vi "HEWH Uniform Energy Factor Minimums.vi"(4 "Maufacturing Date":T7(ring), 7 "Water Heater Type":T6="Gas Storage (Non-Electric)", 8 "error in (no error)":errorcluster, 11 "UEF Calculated Values Input":T1 {"Data Indexes"."15 sec after Draw Index" format="%#.2f"; "Data Indexes"."15 sec after Draw Timestamp" format="%#.2f"; "Data Indexes"."Test Start Timestamp" format="%.2f"; "Data Indexes"."Test End Timestamp" format="%.2f"; "Data Indexes"."T0 Timestamp" format="%.2f"; "Data Indexes"."Tsf Timestamp" format="%.2f"; "Data Indexes"."Tsu0 Timestamp" format="%.2f"; "Data Indexes"."Tmax1 Timestamp" format="%.2f"; "Data Indexes"."Draw Index Timestamp" format="%#.2f"; "Data Indexes"."Non-Draw Timestamp" format="%#.2f"; "Data Indexes"."Heating Timestamp" format="%#.2f"; "Data Indexes"."Start Energy (BTU-Gas)" format="%.6f"; "Data Indexes"."Start Watt Hours" format="%.6f"; "Static Data"."V - Volume of Wh (True)" format="%.5f"; "Static Data"."T-Ambinet Nominal (°F)" format="%.5f"; "Static Data"."T-Inlet Setpoint (°F)" format="%.5f"; "Static Data"."T-Wh Setpoint (°F)" format="%.5f"; "Sampled Data"."Qe (Wh)" format="%.5f"; "Sampled Data"."Tau stby2 (hr)" format="%.5f"; "Sampled Data"."Tastby2 (°F)" format="%.5f"; "Sampled Data"."Qf (BTU)" format="%.5f"; "Sampled Data"."Qe (BTU)" format="%.5f"; "Sampled Data"."Tmax1 (°F)" format="%.5f"; "Sampled Data"."T0 (°F)" format="%.5f"; "Sampled Data"."Qr (BTU)" format="%.5f"; "Sampled Data"."T 24(°F)" format="%.5f"; "Sampled Data"."T astby(°F)" format="%.5f"; "Sampled Data"."T tstby(°F)" format="%.5f"; "Sampled Data"."T su0(°F)" format="%.5f"; "Sampled Data"."T suf(°F)" format="%.5f"; "Sampled Data"."Tau stby_1 (hr)" format="%.5f"; "Sampled Data"."Qsuf (BTU)" format="%.5f"; "Sampled Data"."Qsu0 (BTU)" format="%.5f"; "Calculated Values"."Draw Bonus Volume (gal)" format="%.6f"; "Calculated Values"."Adjustment Factor" format="%.6f"; "Calculated Values"."T*avg_del(n-1)" format="%.6f"; "Calculated Values"."T*min(n-1)" format="%.6f"; "Calculated Values"."T*avg_del(n)" format="%.6f"; "Calculated Values"."Vn" format="%.6f"; "Calculated Values"."Qdm (BTU)" format="%.6f"; "Calculated Values"."QHWD (BTU)" format="%.6f"; "Calculated Values"."QHW (BTU)" format="%.6f"; "Calculated Values"."UEF" format="%.6f"; "Calculated Values"."QHW67 (BTU)" format="%.6f"; "Calculated Values"."Qda (BTU)" format="%.6f"; "Calculated Values"."Qd (BTU)" format="%.6f"; "Calculated Values"."Q (BTU)" format="%.6f"; "Calculated Values"."UA (BTU/(hr*F))" format="%.6f"; "Calculated Values"."Qhr (BTU/hr)" format="%.6f"; "Calculated Values"."Qstby (BTU)" format="%.6f"; "Calculated Values"."nu_r" format="%.6f"; "Calculated Values"."CpUEF (BTU/(lb*F))" format="%.6f"; "Calculated Values"."rho_nu (lb/gal)" format="%.6f"; "Calculated Values"."V1- Vol (Gal)" format="%.6f"; "Calculated Values"."M cluster mass removed (lb)" format="%.6f"; "Calculated Values"."Cp theoretical (BTU/(lbm °F))" format="%.6f"; "Calculated Values"."Tin1 - Mean Inlet 1st Cluster (°F)" format="%.6f"; "Calculated Values"."Tdel1-Mean Outlet 1st Cluster(°F)" format="%.6f"; "Calculated Values"."Cp 24 (BTU/(lb*F))" format="%.6f"; "Calculated Values"."Cp standby (BTU/(lb*F))" format="%.6f"; "Calculated Values"."Cp2 (BTU/(lb*F))" format="%.6f"; "Calculated Values"."Cp1 (BTU/(lb*F))" format="%.6f"; "Calculated Values"."rho 24 (lb/gal)" format="%.6f"; "Calculated Values"."rho standby (lb/gal)" format="%.6f"; "Calculated Values"."rho 2 (lb/gal)" format="%.6f"; "Calculated Values"."Density of cold water All (lbm/gal)" format="%#.3g"; "Calculated Values"."CpHW (BTU/(lbm °F))" format="%#.3g"; "Calculated Values"."Density of hot water All (lbm/gal)" format="%#.3g"; "Calculated Values"."Mass of water All (lbm)" format="%#.3f"}) -> (0 "error out":errorcluster, 3 "UEF Calculated Values Output":T1 {"Data Indexes"."15 sec after Draw Index" format="%#.2f"; "Data Indexes"."15 sec after Draw Timestamp" format="%#.2f"; "Data Indexes"."Test Start Timestamp" format="%.2f"; "Data Indexes"."Test End Timestamp" format="%.2f"; "Data Indexes"."T0 Timestamp" format="%.2f"; "Data Indexes"."Tsf Timestamp" format="%.2f"; "Data Indexes"."Tsu0 Timestamp" format="%.2f"; "Data Indexes"."Tmax1 Timestamp" format="%.2f"; "Data Indexes"."Draw Index Timestamp" format="%#.2f"; "Data Indexes"."Non-Draw Timestamp" format="%#.2f"; "Data Indexes"."Heating Timestamp" format="%#.2f"; "Data Indexes"."Start Energy (BTU-Gas)" format="%.6f"; "Data Indexes"."Start Watt Hours" format="%.6f"; "Static Data"."V - Volume of Wh (True)" format="%.5f"; "Static Data"."T-Ambinet Nominal (°F)" format="%.5f"; "Static Data"."T-Inlet Setpoint (°F)" format="%.5f"; "Static Data"."T-Wh Setpoint (°F)" format="%.5f"; "Sampled Data"."Qe (Wh)" format="%.5f"; "Sampled Data"."Tau stby2 (hr)" format="%.5f"; "Sampled Data"."Tastby2 (°F)" format="%.5f"; "Sampled Data"."Qf (BTU)" format="%.5f"; "Sampled Data"."Qe (BTU)" format="%.5f"; "Sampled Data"."Tmax1 (°F)" format="%.5f"; "Sampled Data"."T0 (°F)" format="%.5f"; "Sampled Data"."Qr (BTU)" format="%.5f"; "Sampled Data"."T 24(°F)" format="%.5f"; "Sampled Data"."T astby(°F)" format="%.5f"; "Sampled Data"."T tstby(°F)" format="%.5f"; "Sampled Data"."T su0(°F)" format="%.5f"; "Sampled Data"."T suf(°F)" format="%.5f"; "Sampled Data"."Tau stby_1 (hr)" format="%.5f"; "Sampled Data"."Qsuf (BTU)" format="%.5f"; "Sampled Data"."Qsu0 (BTU)" format="%.5f"; "Calculated Values"."Draw Bonus Volume (gal)" format="%.6f"; "Calculated Values"."Adjustment Factor" format="%.6f"; "Calculated Values"."T*avg_del(n-1)" format="%.6f"; "Calculated Values"."T*min(n-1)" format="%.6f"; "Calculated Values"."T*avg_del(n)" format="%.6f"; "Calculated Values"."Vn" format="%.6f"; "Calculated Values"."Qdm (BTU)" format="%.6f"; "Calculated Values"."QHWD (BTU)" format="%.6f"; "Calculated Values"."QHW (BTU)" format="%.6f"; "Calculated Values"."UEF" format="%.6f"; "Calculated Values"."QHW67 (BTU)" format="%.6f"; "Calculated Values"."Qda (BTU)" format="%.6f"; "Calculated Values"."Qd (BTU)" format="%.6f"; "Calculated Values"."Q (BTU)" format="%.6f"; "Calculated Values"."UA (BTU/(hr*F))" format="%.6f"; "Calculated Values"."Qhr (BTU/hr)" format="%.6f"; "Calculated Values"."Qstby (BTU)" format="%.6f"; "Calculated Values"."nu_r" format="%.6f"; "Calculated Values"."CpUEF (BTU/(lb*F))" format="%.6f"; "Calculated Values"."rho_nu (lb/gal)" format="%.6f"; "Calculated Values"."V1- Vol (Gal)" format="%.6f"; "Calculated Values"."M cluster mass removed (lb)" format="%.6f"; "Calculated Values"."Cp theoretical (BTU/(lbm °F))" format="%.6f"; "Calculated Values"."Tin1 - Mean Inlet 1st Cluster (°F)" format="%.6f"; "Calculated Values"."Tdel1-Mean Outlet 1st Cluster(°F)" format="%.6f"; "Calculated Values"."Cp 24 (BTU/(lb*F))" format="%.6f"; "Calculated Values"."Cp standby (BTU/(lb*F))" format="%.6f"; "Calculated Values"."Cp2 (BTU/(lb*F))" format="%.6f"; "Calculated Values"."Cp1 (BTU/(lb*F))" format="%.6f"; "Calculated Values"."rho 24 (lb/gal)" format="%.6f"; "Calculated Values"."rho standby (lb/gal)" format="%.6f"; "Calculated Values"."rho 2 (lb/gal)" format="%.6f"; "Calculated Values"."Density of cold water All (lbm/gal)" format="%#.3g"; "Calculated Values"."CpHW (BTU/(lbm °F))" format="%#.3g"; "Calculated Values"."Density of hot water All (lbm/gal)" format="%#.3g"; "Calculated Values"."Mass of water All (lbm)" format="%#.3f"})   [LabVIEW 2023]
uses:
  Type Definitions/HEWH Water Heater Type.ctl
  Type Definitions/UEF Constants.ctl
  Type Definitions/HEWH Draw Stats.ctl
  Type Definitions/HEWH FHR Draw Type.ctl
  Type Definitions/FHR Bins.ctl
  Type Definitions/HEWH Meter Type.ctl
panel:
  # "FHR"
  # "FHR"
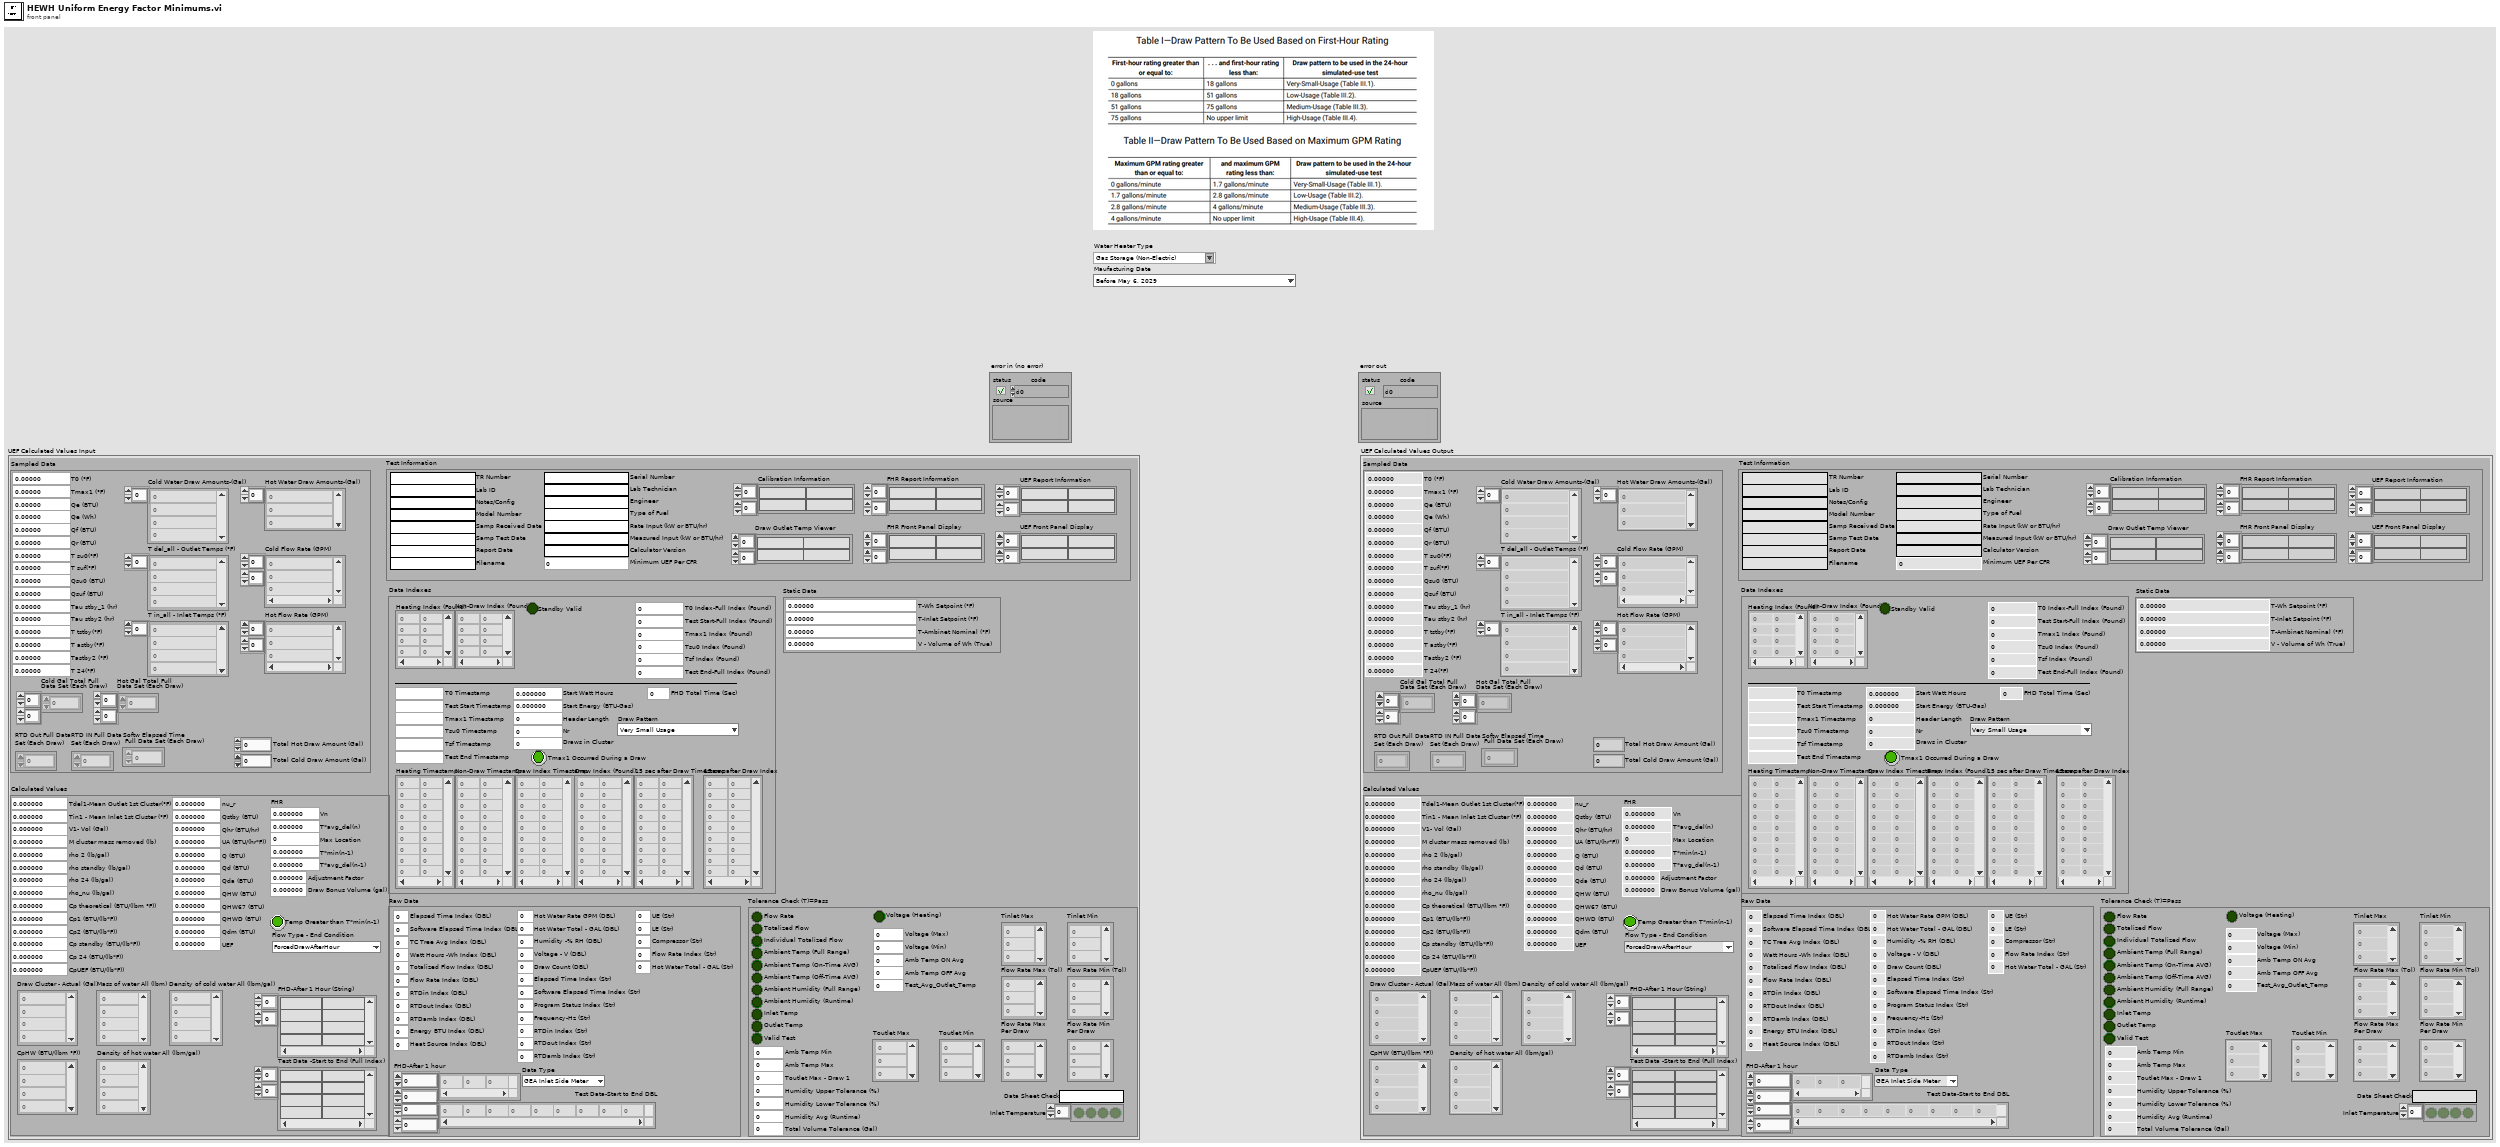
[diagram p1: front panel]
types:
  T1 = typedef "UEF Constants.ctl" = cluster{"Calculated Values":T2, "Sampled Data":cluster{"Cold Water Draw Amounts-(Gal)":dbl[], "T del_all - Outlet Temps (°F)":dbl[], "T in_all - Inlet Temps (°F)":dbl[], "Qsu0 (BTU)":dbl, "Qsuf (BTU)":dbl, "Tau stby_1 (hr)":dbl, "T suf(°F)":dbl, "T su0(°F)":dbl, "T tstby(°F)":dbl, "T astby(°F)":dbl, "T 24(°F)":dbl, "Qr (BTU)":dbl, "T0 (°F)":dbl, "Tmax1 (°F)":dbl, "Qe (BTU)":dbl, "Qf (BTU)":dbl, "Tastby2 (°F)":dbl, "RTD Out Full Data\nSet (Each Draw)":dbl[][], "RTD IN Full Data\nSet (Each Draw)":dbl[][], "Tau stby2 (hr)":dbl, "Hot Water Draw Amounts-(Gal)":dbl[], "Cold Flow Rate (GPM)":dbl[][], "Hot Flow Rate (GPM)":dbl[][], "Softw Elapsed Time\n Full Data Set (Each Draw)":dbl[][], "Cold Gal Total Full\nData Set (Each Draw)":dbl[][], "Total Hot Draw Amount (Gal) ":dbl, "Total Cold Draw Amount (Gal)":dbl, "Qe (Wh)":dbl, "Hot Gal Total Full\nData Set (Each Draw)":dbl[][]}, "Static Data":cluster{"T-Wh Setpoint (°F)":dbl, "T-Inlet Setpoint (°F)":dbl, "T-Ambinet Nominal (°F)":dbl, "V - Volume of Wh (True)":dbl}, "Data Indexes":cluster{"Test Start-Full Index (Found)":i32, "Header Length":i32, "Draw Index (Found)":i32[][], "Nr":i32, "Start Watt Hours":dbl, "Tsu0 Index (Found)":i32, "Tsf Index (Found)":i32, "Start Energy (BTU-Gas)":dbl, "Draws in Cluster":i32, "T0 Index-Full Index (Found)":i32, "Non-Draw Index (Found)":i32[][], "Tmax1 Index (Found)":i32, "Test End-Full Index (Found)":i32, "Heating Index (Found)":i32[][], "Heating Timestamp":dbl[][], "Non-Draw Timestamp":dbl[][], "Draw Index Timestamp":dbl[][], "Tmax1 Timestamp":dbl, "Tsu0 Timestamp":dbl, "Tsf Timestamp":dbl, "T0 Timestamp":dbl, "Test End Timestamp":dbl, "Test Start Timestamp":dbl, "15 sec after Draw Timestamp":dbl[][], "15 sec after Draw Index":dbl[][], "Tmax1 Occurred During a Draw":bool, "FHD Total Time (Sec)":dbl, "Draw Pattern":T4, "Standby Valid":bool}, "Raw Data":cluster{"Elapsed Time Index (DBL)":i32, "Software Elapsed Time Index (DBL)":i32, "TC Tree Avg Index (DBL)":i32, "Watt Hours -Wh Index (DBL)":i32, "Energy BTU Index (DBL)":i32, "Totalized Flow Index (DBL)":i32, "Flow Rate Index (DBL)":i32, "Program Status Index (Str)":i32, "RTDin Index (DBL)":i32, "RTDout Index (DBL)":i32, "RTDamb Index (DBL)":i32, "Test Data-Start to End DBL":dbl[][], "Data Type":T5, "Heat Source Index (DBL)":i32, "Hot Water Rate GPM (DBL)":i32, "Hot Water Total - GAL (DBL)":i32, "FHD-After 1 hour":dbl[][], "Humidity -% RH (DBL)":i32, "Voltage - V (DBL)":i32, "Draw Count (DBL)":i32, "Elapsed Time Index (Str)":i32, "Software Elapsed Time Index (Str)":i32, "Frequency-Hz (Str)":i32, "RTDin Index (Str)":i32, "RTDout Index (Str)":i32, "RTDamb Index (Str)":i32, "UE (Str)":i32, "LE (Str)":i32, "Compressor (Str)":i32, "Flow Rate Index (Str)":i32, "Hot Water Total - GAL (Str)":i32}, "Tolerance Check (T)=Pass":cluster{"Flow Rate":bool, "Totalized Flow":bool, "Ambient Temp (Full Range)":bool, "Ambient Humidity (Full Range)":bool, "Inlet Temp":bool, "Outlet Temp":bool, "Valid Test":bool, "Individual Totalized Flow":bool, "Data Sheet Check":string, "Inlet Temperature":bool[], "Tinlet Max":dbl[], "Tinlet Min":dbl[], "Flow Rate Max (Tol)":dbl[], "Flow Rate Min (Tol)":dbl[], "Amb Temp Max":dbl, "Amb Temp Min":dbl, "Toutlet Max - Draw 1":dbl, "Humidity Upper Tolerance (%)":dbl, "Total Volume Tolerance (Gal)":dbl, "Humidity Lower Tolerance (%)":dbl, "Flow Rate Max\nPer Draw":dbl[], "Flow Rate Min\nPer Draw":dbl[], "Ambient Humidity (Runtime)":bool, "Humidity Avg (Runtime)":dbl, "Ambient Temp (On-Time AVG)":bool, "Ambient Temp (Off-Time AVG)":bool, "Amb Temp OFF Avg":dbl, "Amb Temp ON Avg":dbl, "Voltage (Heating)":bool, "Voltage (Min)":dbl, "Voltage (Max)":dbl, "Toutlet Max":dbl[], "Toutlet Min":dbl[], "Test_Avg_Outlet_Temp":dbl}, "Test Information":cluster{"TR Number":string, "Lab ID":string, "Notes/Config":string, "Model Number":string, "Serial Number":string, "Lab Technician":string, "Engineer":string, "Type of Fuel":string, "Samp Received Date":string, "Samp Test Date":string, "Report Date":string, "Rate Input (kW or BTU/hr)":string, "Measured Input (kW or BTU/hr)":string, "Filename":string, "Calibration Information":string[][], "Calculator Version":string, "Minimum UEF Per CFR":dbl, "UEF Report Information":string[][], "FHR Report Information":string[][], "FHR Front Panel Display":string[][], "UEF Front Panel Display":string[][], "Draw Outlet Temp Viewer":string[][]}}
  T2 = typedef "HEWH Draw Stats.ctl" = cluster{"Draw Cluster - Actual (Gal)":dbl[], "Mass of water All (lbm)":dbl[], "Density of hot water All (lbm/gal)":dbl[], "CpHW (BTU/(lbm °F))":dbl[], "rho 2 (lb/gal)":dbl, "rho standby (lb/gal)":dbl, "rho 24 (lb/gal)":dbl, "Cp1 (BTU/(lb*F))":dbl, "Cp2 (BTU/(lb*F))":dbl, "Cp standby (BTU/(lb*F))":dbl, "Cp 24 (BTU/(lb*F))":dbl, "nu_r":dbl, "Qstby (BTU)":dbl, "Qhr (BTU/hr)":dbl, "UA (BTU/(hr*F))":dbl, "Q (BTU)":dbl, "Qd (BTU)":dbl, "Qda (BTU)":dbl, "QHW67 (BTU)":dbl, "UEF":dbl, "Tdel1-Mean Outlet 1st Cluster(°F)":dbl, "Tin1 - Mean Inlet 1st Cluster (°F)":dbl, "Cp theoretical (BTU/(lbm °F))":dbl, "M cluster mass removed (lb)":dbl, "V1- Vol (Gal)":dbl, "Test Data -Start to End (Full Index)":string[][], "rho_nu (lb/gal)":dbl, "Density of cold water All (lbm/gal)":dbl[], "CpUEF (BTU/(lb*F))":dbl, "QHW (BTU)":dbl, "QHWD (BTU)":dbl, "Qdm (BTU)":dbl, "FHD-After 1 Hour (String)":string[][], "Vn":dbl, "T*avg_del(n)":dbl, "Max Location":i32, "T*min(n-1)":dbl, "T*avg_del(n-1)":dbl, "Temp Greater than T*min(n-1)":bool, "Adjustment Factor":dbl, "Draw Bonus Volume (gal)":dbl, "Flow Type - End Condition":T3}
  T3 = typedef "HEWH FHR Draw Type.ctl" = enum16{"ForcedDrawAfterHour", "HeatingCutoffBeforeHour"}
  T4 = typedef "FHR Bins.ctl" = enum16{"Very Small Usage", "Low Usage", "Medium Usage", "High Usage", "Undefined"}
  T5 = typedef "HEWH Meter Type.ctl" = enum16{"GEA Inlet Side Meter", "GEA Outlet Side Meter", "CSA Inlet Side Meter"}
  T6 = typedef "HEWH Water Heater Type.ctl" = string
  T7 = enum16{"Before May 6, 2029", "On or After May 6, 2029"}
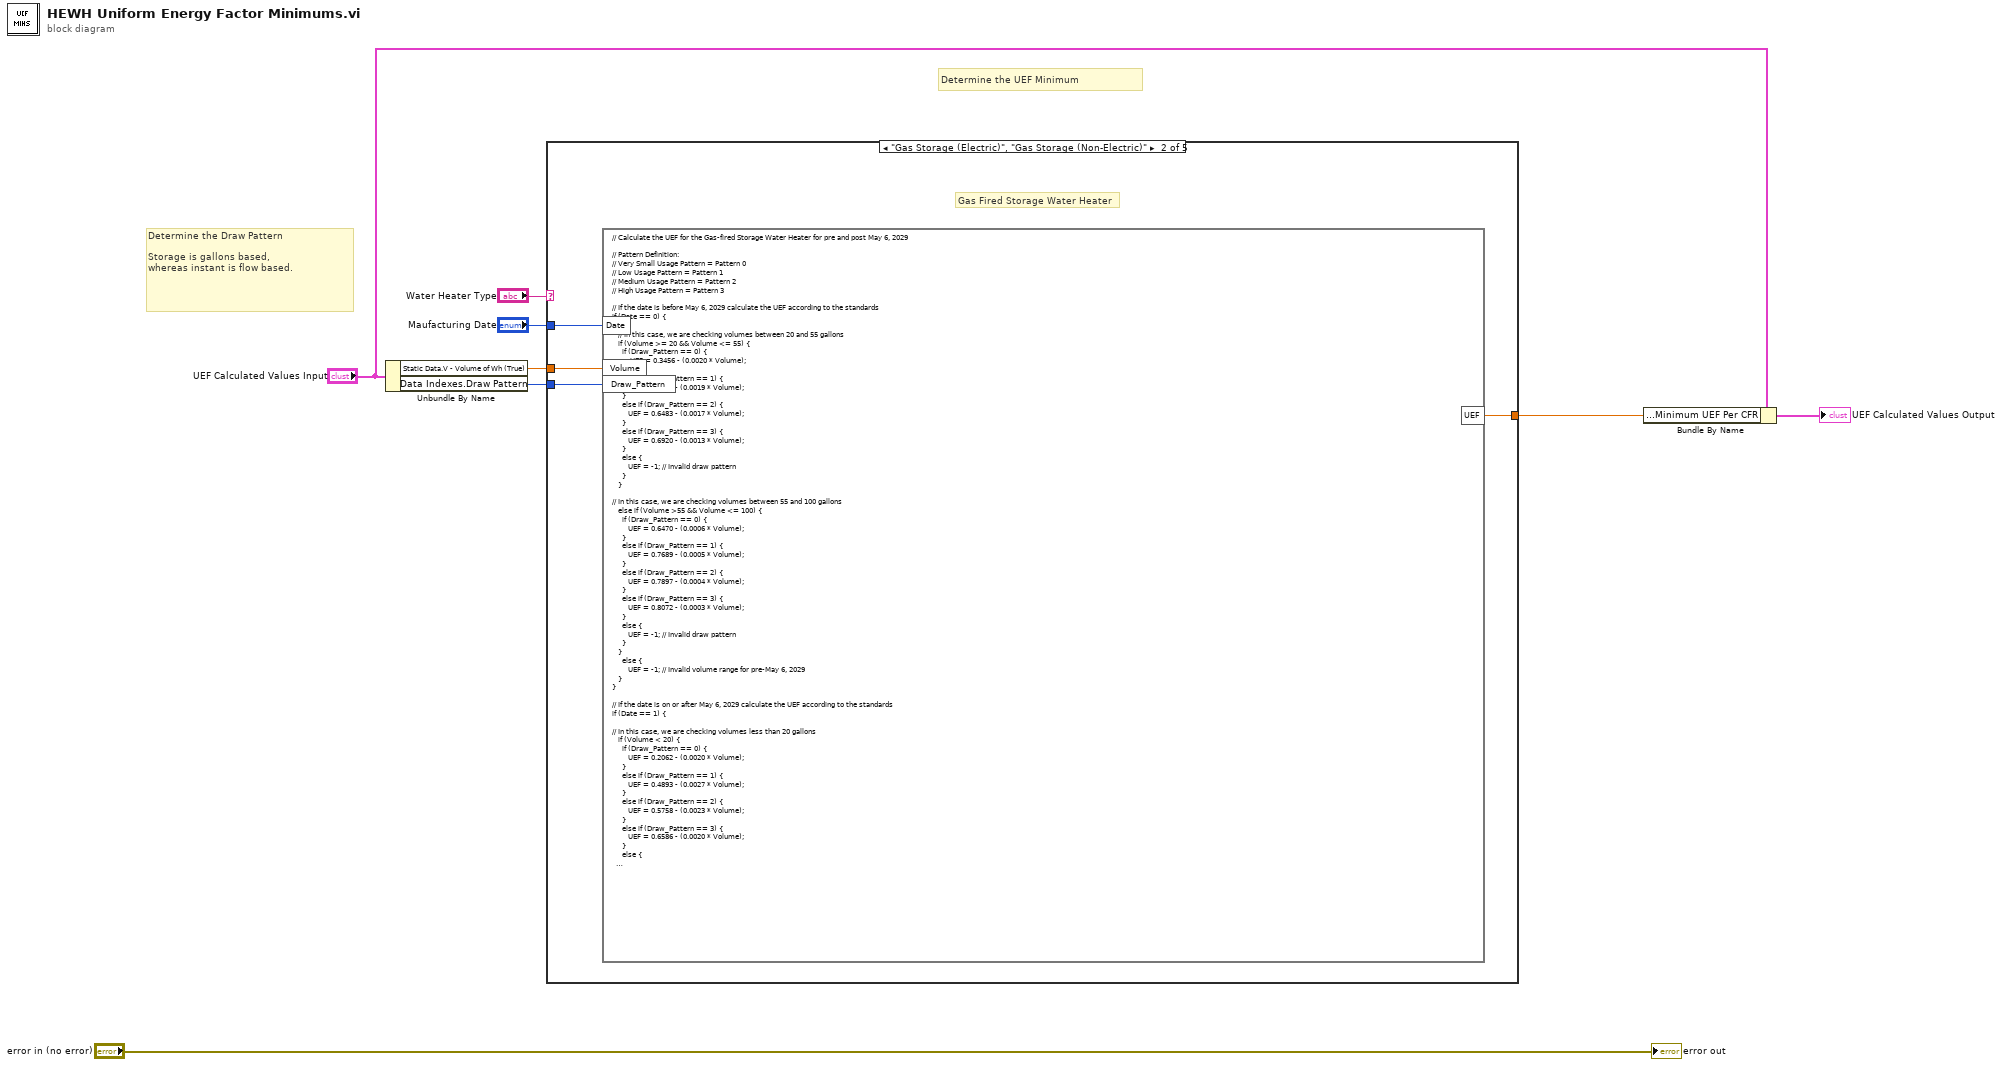
[diagram p0: block diagram]
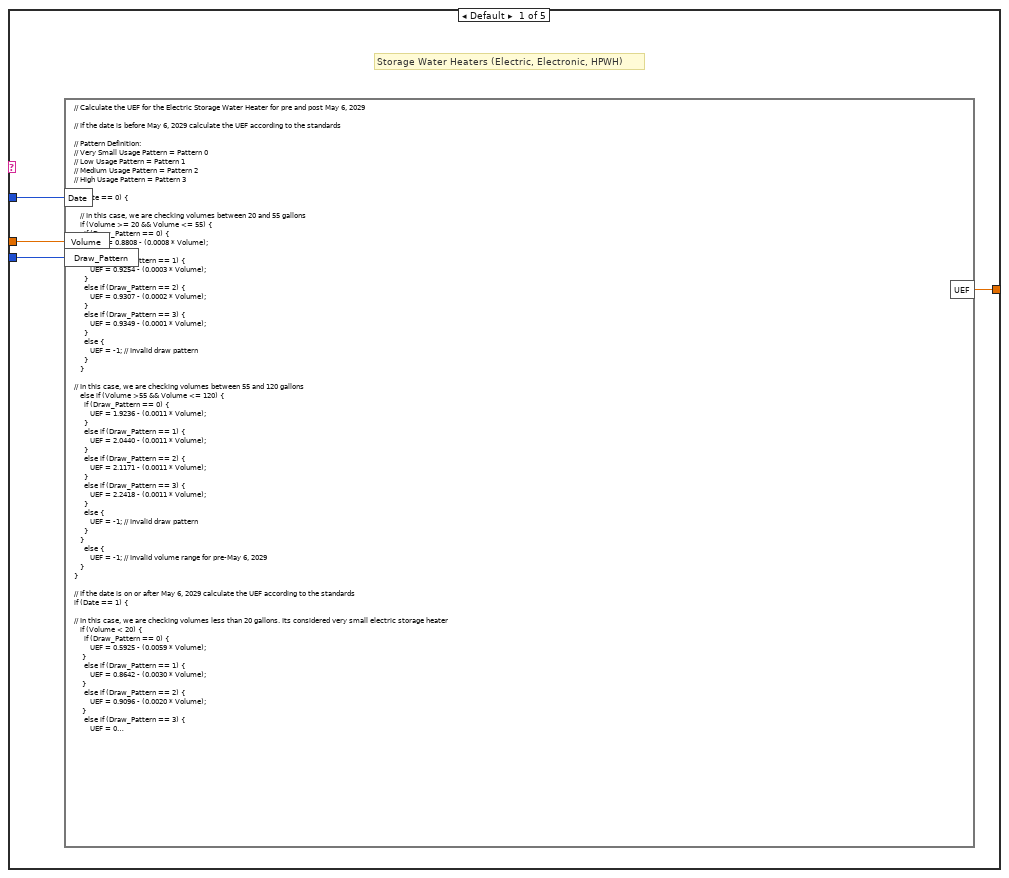
[diagram p2: hidden frame]
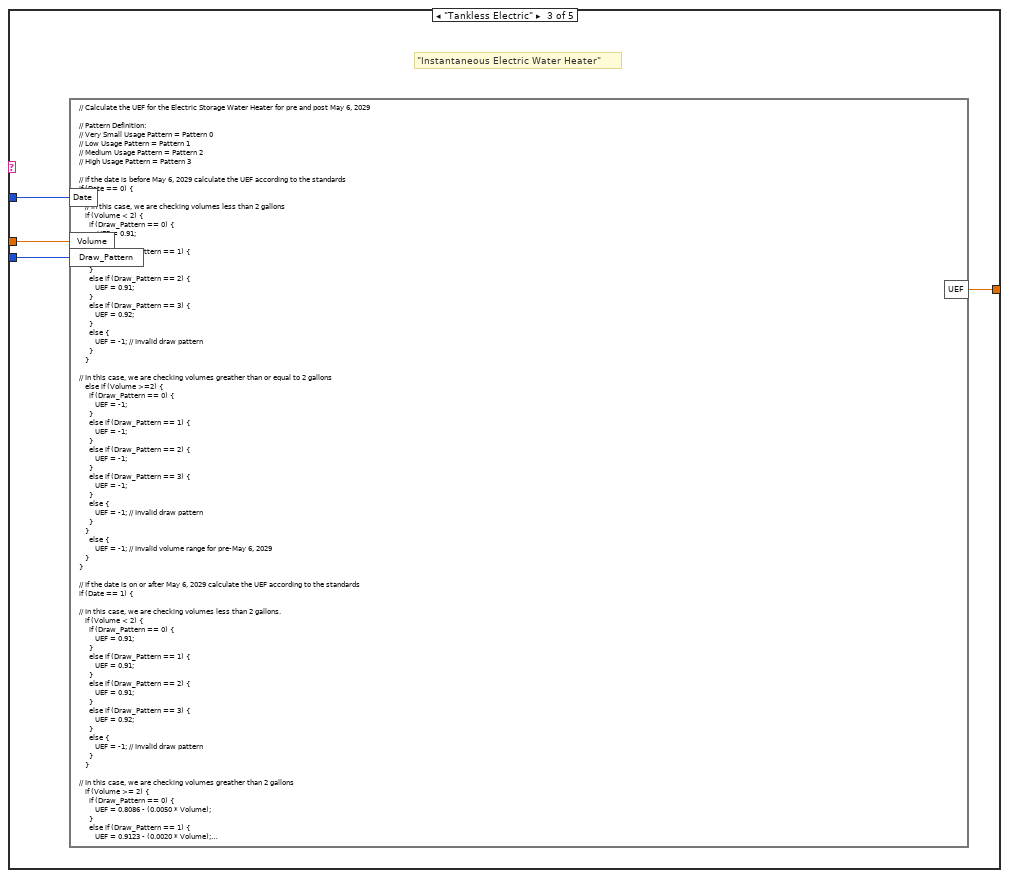
[diagram p3: hidden frame]
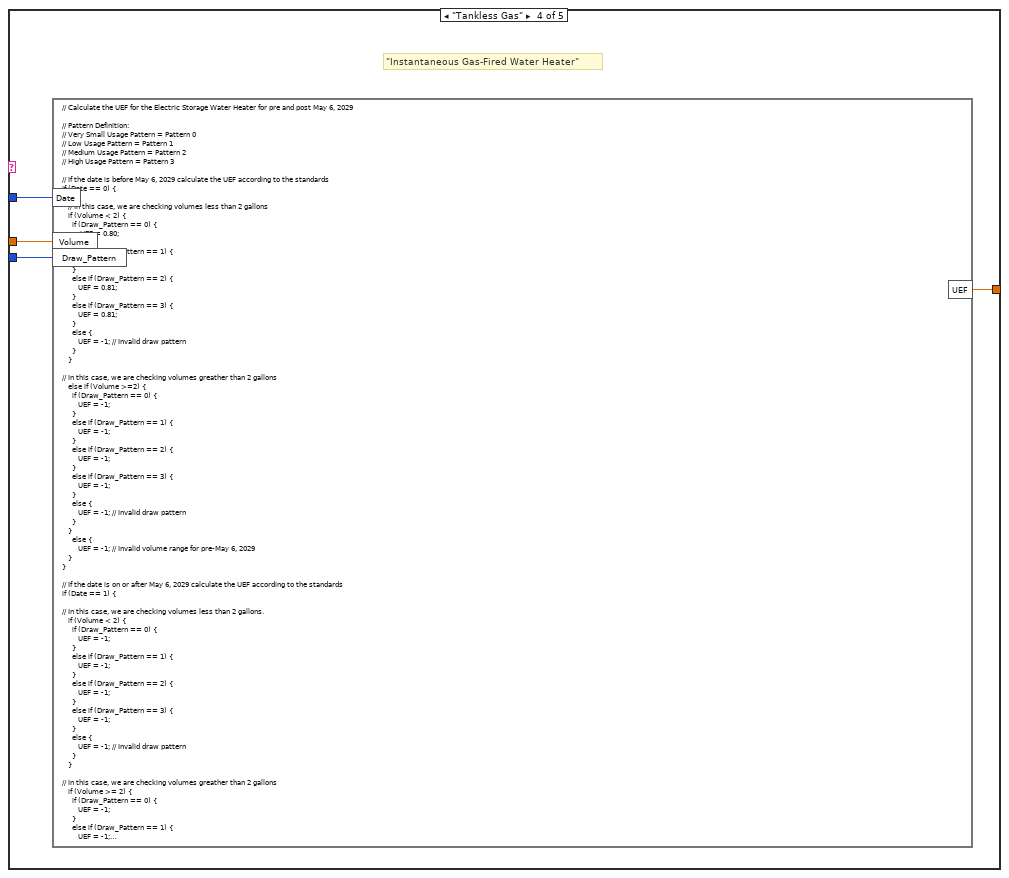
[diagram p4: hidden frame]
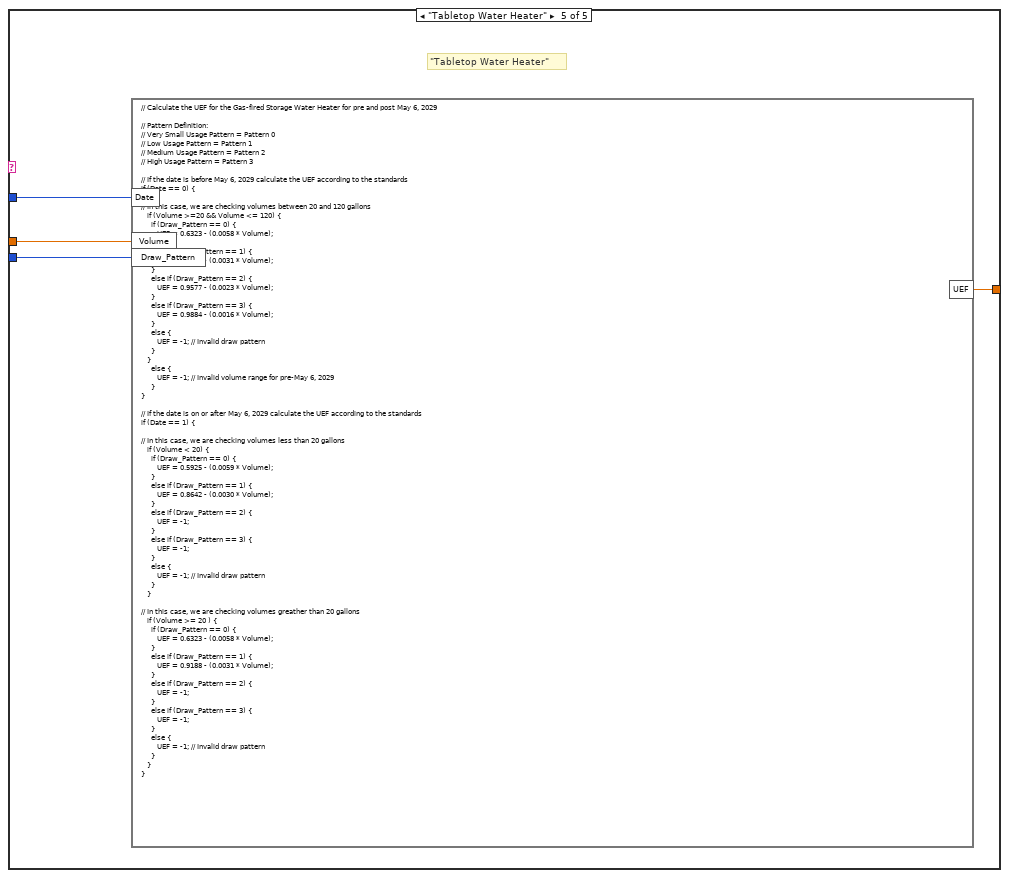
[diagram p5: hidden frame]
diagram:
  # "Determine the UEF Minimum"
  # "Determine the Draw Pattern\n\nStorage is gallons based,\nwhereas instant is flow based."
  n1 = Unbundle By Name("UEF Calculated Values Input") -> ("Static Data.V - Volume of Wh (True)"=w6:dbl, "Data Indexes.Draw Pattern"=w4:T4)
  n2 = case shown="\"Gas Storage (Electric)\", \"Gas Storage (Non-Electric)\"" "Water Heater Type" {
    tunnel: w6 -> [w9 w16 w19 w23 w27]
    tunnel: w4 -> [w10 w15 w18 w22 w26]
    tunnel: [w12 w14 w20 w24 w28] -> w1
    tunnel: "Maufacturing Date" -> [w11 w13 w17 w21 w25]
    frame Default {
      # "Storage Water Heaters (Electric, Electronic, HPWH)"
      n3 = formula code="// Calculate the UEF for the Electric Storage Water Heater for pre and post May 6, 2029\n\n// If the date is before May 6, 2029 calculate the UEF according to the standards\n\n// Pattern Definition:\n// Very Small Usage Pattern = Pattern 0\n// Low Usage Pattern = Pattern 1\n// Medium Usage Pattern = Pattern 2\n// High Usage Pattern = Pattern 3\n\nif (Date == 0) {\n\n   // In this case, we are checking volumes between 20 and 55 gallons\n   if (Volume >= 20 && Volume <= 55) {\n     if (Draw_Pattern == 0) {\n         UEF = 0.8808 - (0.0008 * Volume);\n     } \n     else if (Draw_Pattern == 1) {\n        UEF = 0.9254 - (0.0003 * Volume);\n     } \n     else if (Draw_Pattern == 2) {\n        UEF = 0.9307 - (0.0002 * Volume);\n     } \n     else if (Draw_Pattern == 3) {\n        UEF = 0.9349 - (0.0001 * Volume);\n     }\n     else {\n        UEF = -1; // Invalid draw pattern\n     }\n   } \n\n// In this case, we are checking volumes between 55 and 120 gallons\n   else if (Volume >55 && Volume <= 120) {\n     if (Draw_Pattern == 0) {\n        UEF = 1.9236 - (0.0011 * Volume);\n     } \n     else if (Draw_Pattern == 1) {\n        UEF = 2.0440 - (0.0011 * Volume);\n     } \n     else if (Draw_Pattern == 2) {\n        UEF = 2.1171 - (0.0011 * Volume);\n     } \n     else if (Draw_Pattern == 3) {\n        UEF = 2.2418 - (0.0011 * Volume);\n     }\n     else {\n        UEF = -1; // Invalid draw pattern\n     }\n   }\n     else {\n        UEF = -1; // Invalid volume range for pre-May 6, 2029\n   } \n}\n\n// If the date is on or after May 6, 2029 calculate the UEF according to the standards\nif (Date == 1) {\n\n// In this case, we are checking volumes less than 20 gallons. Its considered very small electric storage heater\n   if (Volume < 20) {\n     if (Draw_Pattern == 0) {\n        UEF = 0.5925 - (0.0059 * Volume);\n    } \n     else if (Draw_Pattern == 1) {\n        UEF = 0.8642 - (0.0030 * Volume);\n    } \n     else if (Draw_Pattern == 2) {\n        UEF = 0.9096 - (0.0020 * Volume);\n    } \n     else if (Draw_Pattern == 3) {\n        UEF = 0.9430 - (0.0012 * Volume);\n    }\n     else {\n        UEF = -1; // Invalid draw pattern\n    }\n}\n\n// In this case, we are checking volumes between 20 and 55 gallons, not considered small electric water heater)\n   if (Volume >= 20 && Volume <= 55) {\n     if (Draw_Pattern == 0) {\n        UEF = 2.30;\n    } \n     else if (Draw_Pattern == 1) {\n        UEF = 2.30;\n    } \n     else if (Draw_Pattern == 2) {\n        UEF = 2.30;\n    } \n     else if (Draw_Pattern == 3) {\n        UEF = 2.30;\n    }\n     else {\n        UEF = -1; // Invalid draw pattern\n    }\n} \n\n// In this case, we are checking volumes between 55 and 120 gallons\n   if (Volume >55 && Volume <= 120) {\n     if (Draw_Pattern == 0) {\n        UEF = 2.50;\n    } \n     else if (Draw_Pattern == 1) {\n        UEF = 2.50;\n    } \n     else if (Draw_Pattern == 2) {\n        UEF = 2.50;\n    } \n     else if (Draw_Pattern == 3) {\n        UEF = 2.50;\n    }\n     else {\n        UEF = -1; // Invalid draw pattern\n    }\n} \n\n// In this case, we are checking volumes greater than 120 gallons\n   if (Volume > 120) {\n     if (Draw_Pattern == 0) {\n        UEF = 0.3574 - (0.0012 * Volume);\n    } \n     else if (Draw_Pattern == 1) {\n        UEF = 0.7897 - (0.0019 * Volume);\n    } \n     else if (Draw_Pattern == 2) {\n        UEF = 0.8884 - (0.0017 * Volume);\n    } \n     else if (Draw_Pattern == 3) {\n        UEF = 0.9575 - (0.0013 * Volume);\n    }\n     else {\n        UEF = -1; // Invalid draw pattern\n    }\n}\n}"("Volume"=w9, "Draw_Pattern"=w10, "Date"=w11) -> ("UEF"=w12:dbl)
    }
    frame "Gas Storage (Electric)", "Gas Storage (Non-Electric)" {
      # "Gas Fired Storage Water Heater"
      n4 = formula code="// Calculate the UEF for the Gas-fired Storage Water Heater for pre and post May 6, 2029\n\n// Pattern Definition:\n// Very Small Usage Pattern = Pattern 0\n// Low Usage Pattern = Pattern 1\n// Medium Usage Pattern = Pattern 2\n// High Usage Pattern = Pattern 3\n\n// If the date is before May 6, 2029 calculate the UEF according to the standards\nif (Date == 0) {\n\n   // In this case, we are checking volumes between 20 and 55 gallons\n   if (Volume >= 20 && Volume <= 55) {\n     if (Draw_Pattern == 0) {\n         UEF = 0.3456 - (0.0020 * Volume);\n     } \n     else if (Draw_Pattern == 1) {\n        UEF = 0.5982 - (0.0019 * Volume);\n     } \n     else if (Draw_Pattern == 2) {\n        UEF = 0.6483 - (0.0017 * Volume);\n     } \n     else if (Draw_Pattern == 3) {\n        UEF = 0.6920 - (0.0013 * Volume);\n     }\n     else {\n        UEF = -1; // Invalid draw pattern\n     }\n   } \n\n// In this case, we are checking volumes between 55 and 100 gallons\n   else if (Volume >55 && Volume <= 100) {\n     if (Draw_Pattern == 0) {\n        UEF = 0.6470 - (0.0006 * Volume);\n     } \n     else if (Draw_Pattern == 1) {\n        UEF = 0.7689 - (0.0005 * Volume);\n     } \n     else if (Draw_Pattern == 2) {\n        UEF = 0.7897 - (0.0004 * Volume);\n     } \n     else if (Draw_Pattern == 3) {\n        UEF = 0.8072 - (0.0003 * Volume);\n     }\n     else {\n        UEF = -1; // Invalid draw pattern\n     }\n   }\n     else {\n        UEF = -1; // Invalid volume range for pre-May 6, 2029\n   } \n}\n\n// If the date is on or after May 6, 2029 calculate the UEF according to the standards\nif (Date == 1) {\n\n// In this case, we are checking volumes less than 20 gallons\n   if (Volume < 20) {\n     if (Draw_Pattern == 0) {\n        UEF = 0.2062 - (0.0020 * Volume);\n     } \n     else if (Draw_Pattern == 1) {\n        UEF = 0.4893 - (0.0027 * Volume);\n     } \n     else if (Draw_Pattern == 2) {\n        UEF = 0.5758 - (0.0023 * Volume);\n     } \n     else if (Draw_Pattern == 3) {\n        UEF = 0.6586 - (0.0020 * Volume);\n     }\n     else {\n        UEF = -1; // Invalid draw pattern\n     }\n   }\n\n// In this case, we are checking volumes between 20 and 55 gallons\n   if (Volume >= 20 && Volume <= 55) {\n     if (Draw_Pattern == 0) {\n        UEF = 0.3925 - (0.0020 * Volume);\n     } \n     else if (Draw_Pattern == 1) {\n        UEF = 0.6451 - (0.0019 * Volume);\n     } \n     else if (Draw_Pattern == 2) {\n        UEF = 0.7046 - (0.0017 * Volume);\n     } \n     else if (Draw_Pattern == 3) {\n        UEF = 0.7424 - (0.0013 * Volume);\n     }\n     else {\n        UEF = -1; // Invalid draw pattern\n     }\n   } \n\n// In this case, we are checking volumes between 55 and 100 gallons\n   if (Volume >55 && Volume <= 100) {\n     if (Draw_Pattern == 0) {\n        UEF = 0.6470 - (0.0006 * Volume);\n     } \n     else if (Draw_Pattern == 1) {\n        UEF = 0.7689 - (0.0005 * Volume);\n     } \n     else if (Draw_Pattern == 2) {\n        UEF = 0.7897 - (0.0004 * Volume);\n     } \n     else if (Draw_Pattern == 3) {\n        UEF = 0.8072 - (0.0003 * Volume);\n     }\n     else {\n        UEF = -1; // Invalid draw pattern\n     }\n   } \n\n// In this case, we are checking volumes greater than 100 gallons\n   if (Volume > 100) {\n     if (Draw_Pattern == 0) {\n        UEF = 0.1482 - (0.0007 * Volume);\n     } \n     else if (Draw_Pattern == 1) {\n        UEF = 0.4342 - (0.0017 * Volume);\n     } \n     else if (Draw_Pattern == 2) {\n        UEF = 0.5596 - (0.0020 * Volume);\n     } \n     else if (Draw_Pattern == 3) {\n        UEF = 0.6658 - (0.0019 * Volume);\n     }\n     else {\n        UEF = -1; // Invalid draw pattern\n     }\n   }\n}"("Volume"=w16, "Draw_Pattern"=w15, "Date"=w13) -> ("UEF"=w14:dbl)
    }
    frame "Tankless Electric" {
      # "\"Instantaneous Electric Water Heater\""
      n5 = formula code="// Calculate the UEF for the Electric Storage Water Heater for pre and post May 6, 2029\n\n// Pattern Definition:\n// Very Small Usage Pattern = Pattern 0\n// Low Usage Pattern = Pattern 1\n// Medium Usage Pattern = Pattern 2\n// High Usage Pattern = Pattern 3\n\n// If the date is before May 6, 2029 calculate the UEF according to the standards\nif (Date == 0) {\n\n   // In this case, we are checking volumes less than 2 gallons\n   if (Volume < 2) {\n     if (Draw_Pattern == 0) {\n         UEF = 0.91;\n     } \n     else if (Draw_Pattern == 1) {\n        UEF = 0.91;\n     } \n     else if (Draw_Pattern == 2) {\n        UEF = 0.91;\n     } \n     else if (Draw_Pattern == 3) {\n        UEF = 0.92;\n     }\n     else {\n        UEF = -1; // Invalid draw pattern\n     }   \n   } \n\n// In this case, we are checking volumes greather than or equal to 2 gallons\n   else if (Volume >=2) {\n     if (Draw_Pattern == 0) {\n        UEF = -1;\n     } \n     else if (Draw_Pattern == 1) {\n        UEF = -1;\n     } \n     else if (Draw_Pattern == 2) {\n        UEF = -1;\n     } \n     else if (Draw_Pattern == 3) {\n        UEF = -1;\n     }\n     else {\n        UEF = -1; // Invalid draw pattern\n     }\n   }\n     else {\n        UEF = -1; // Invalid volume range for pre-May 6, 2029\n   } \n}\n\n// If the date is on or after May 6, 2029 calculate the UEF according to the standards\nif (Date == 1) {\n\n// In this case, we are checking volumes less than 2 gallons.\n   if (Volume < 2) {\n     if (Draw_Pattern == 0) {\n        UEF = 0.91;\n     } \n     else if (Draw_Pattern == 1) {\n        UEF = 0.91;\n     } \n     else if (Draw_Pattern == 2) {\n        UEF = 0.91;\n     } \n     else if (Draw_Pattern == 3) {\n        UEF = 0.92;\n     }\n     else {\n        UEF = -1; // Invalid draw pattern\n     }\n   }\n\n// In this case, we are checking volumes greather than 2 gallons\n   if (Volume >= 2) {\n     if (Draw_Pattern == 0) {\n        UEF = 0.8086 - (0.0050 * Volume);\n     } \n     else if (Draw_Pattern == 1) {\n        UEF = 0.9123 - (0.0020 * Volume);\n     } \n     else if (Draw_Pattern == 2) {\n        UEF = 0.9252 - (0.0015 * Volume);\n     } \n     else if (Draw_Pattern == 3) {\n        UEF = 0.9350 - (0.0011 * Volume);\n     }\n     else {\n        UEF = -1; // Invalid draw pattern\n     }\n   } \n}"("Volume"=w19, "Draw_Pattern"=w18, "Date"=w17) -> ("UEF"=w20:dbl)
    }
    frame "Tankless Gas" {
      # "\"Instantaneous Gas-Fired Water Heater\""
      n6 = formula code="// Calculate the UEF for the Electric Storage Water Heater for pre and post May 6, 2029\n\n// Pattern Definition:\n// Very Small Usage Pattern = Pattern 0\n// Low Usage Pattern = Pattern 1\n// Medium Usage Pattern = Pattern 2\n// High Usage Pattern = Pattern 3\n\n// If the date is before May 6, 2029 calculate the UEF according to the standards\nif (Date == 0) {\n\n   // In this case, we are checking volumes less than 2 gallons\n   if (Volume < 2) {\n     if (Draw_Pattern == 0) {\n         UEF = 0.80;\n     } \n     else if (Draw_Pattern == 1) {\n        UEF = 0.81;\n     } \n     else if (Draw_Pattern == 2) {\n        UEF = 0.81;\n     } \n     else if (Draw_Pattern == 3) {\n        UEF = 0.81;\n     }\n     else {\n        UEF = -1; // Invalid draw pattern\n     }\n   } \n\n// In this case, we are checking volumes greather than 2 gallons\n   else if (Volume >=2) {\n     if (Draw_Pattern == 0) {\n        UEF = -1;\n     } \n     else if (Draw_Pattern == 1) {\n        UEF = -1;\n     } \n     else if (Draw_Pattern == 2) {\n        UEF = -1;\n     } \n     else if (Draw_Pattern == 3) {\n        UEF = -1;\n     }\n     else {\n        UEF = -1; // Invalid draw pattern\n     }\n   }\n     else {\n        UEF = -1; // Invalid volume range for pre-May 6, 2029\n   } \n}\n\n// If the date is on or after May 6, 2029 calculate the UEF according to the standards\nif (Date == 1) {\n\n// In this case, we are checking volumes less than 2 gallons.\n   if (Volume < 2) {\n     if (Draw_Pattern == 0) {\n        UEF = -1;\n     } \n     else if (Draw_Pattern == 1) {\n        UEF = -1;\n     } \n     else if (Draw_Pattern == 2) {\n        UEF = -1;\n     } \n     else if (Draw_Pattern == 3) {\n        UEF = -1;\n     }\n     else {\n        UEF = -1; // Invalid draw pattern\n     }\n   }\n\n// In this case, we are checking volumes greather than 2 gallons\n   if (Volume >= 2) {\n     if (Draw_Pattern == 0) {\n        UEF = -1;\n     } \n     else if (Draw_Pattern == 1) {\n        UEF = -1;\n     } \n     else if (Draw_Pattern == 2) {\n        UEF = -1;\n     } \n     else if (Draw_Pattern == 3) {\n        UEF = -1;\n     }\n     else {\n        UEF = -1; // Invalid draw pattern\n     }\n   } \n}"("Volume"=w23, "Draw_Pattern"=w22, "Date"=w21) -> ("UEF"=w24:dbl)
    }
    frame "Tabletop Water Heater" {
      # "\"Tabletop Water Heater\""
      n7 = formula code="// Calculate the UEF for the Gas-fired Storage Water Heater for pre and post May 6, 2029\n\n// Pattern Definition:\n// Very Small Usage Pattern = Pattern 0\n// Low Usage Pattern = Pattern 1\n// Medium Usage Pattern = Pattern 2\n// High Usage Pattern = Pattern 3\n\n// If the date is before May 6, 2029 calculate the UEF according to the standards\nif (Date == 0) {\n\n// In this case, we are checking volumes between 20 and 120 gallons\n   if (Volume >=20 && Volume <= 120) {\n     if (Draw_Pattern == 0) {\n        UEF = 0.6323 - (0.0058 * Volume);\n     } \n     else if (Draw_Pattern == 1) {\n        UEF = 0.9188 - (0.0031 * Volume);\n     } \n     else if (Draw_Pattern == 2) {\n        UEF = 0.9577 - (0.0023 * Volume);\n     } \n     else if (Draw_Pattern == 3) {\n        UEF = 0.9884 - (0.0016 * Volume);\n     }\n     else {\n        UEF = -1; // Invalid draw pattern\n     }\n   }\n     else {\n        UEF = -1; // Invalid volume range for pre-May 6, 2029\n     } \n}\n\n// If the date is on or after May 6, 2029 calculate the UEF according to the standards\nif (Date == 1) {\n\n// In this case, we are checking volumes less than 20 gallons\n   if (Volume < 20) {\n     if (Draw_Pattern == 0) {\n        UEF = 0.5925 - (0.0059 * Volume);\n     } \n     else if (Draw_Pattern == 1) {\n        UEF = 0.8642 - (0.0030 * Volume);\n     } \n     else if (Draw_Pattern == 2) {\n        UEF = -1;\n     } \n     else if (Draw_Pattern == 3) {\n        UEF = -1;\n     }\n     else {\n        UEF = -1; // Invalid draw pattern\n     }\n   }\n\n// In this case, we are checking volumes greather than 20 gallons\n   if (Volume >= 20 ) {\n     if (Draw_Pattern == 0) {\n        UEF = 0.6323 - (0.0058 * Volume);\n     } \n     else if (Draw_Pattern == 1) {\n        UEF = 0.9188 - (0.0031 * Volume);\n     } \n     else if (Draw_Pattern == 2) {\n        UEF = -1;\n     } \n     else if (Draw_Pattern == 3) {\n        UEF = -1;\n     }\n     else {\n        UEF = -1; // Invalid draw pattern\n     }\n   } \n}"("Volume"=w27, "Draw_Pattern"=w26, "Date"=w25) -> ("UEF"=w28:dbl)
    }
  }
  n8 = Bundle By Name(cluster="UEF Calculated Values Input", "Test Information.Minimum UEF Per CFR"=w1) -> (→"UEF Calculated Values Output":T1)
  "error out" <- "error in (no error)"
